vi "设置界面.vi"() -> ()   [LabVIEW 2016, in "DGUS.lvlib"]
uses:
  DGUS.lvlib
  <vilib>/Utility/config.llb/NI_LVConfig.lvlib
panel:
  in  "小数位":u16=2
  in  "底图":enum16{"常规", "摄氏度"}(ring)
  in  "单位":string
  in  "英文名称":string
  in  "中文名称":string
  in  "底部标题":string
  in  "保存按钮":bool
  in  "删除按钮":bool
  in  "添加按钮":bool
  in  "参数列表":i32(listbox)
  # "显示信息设置"
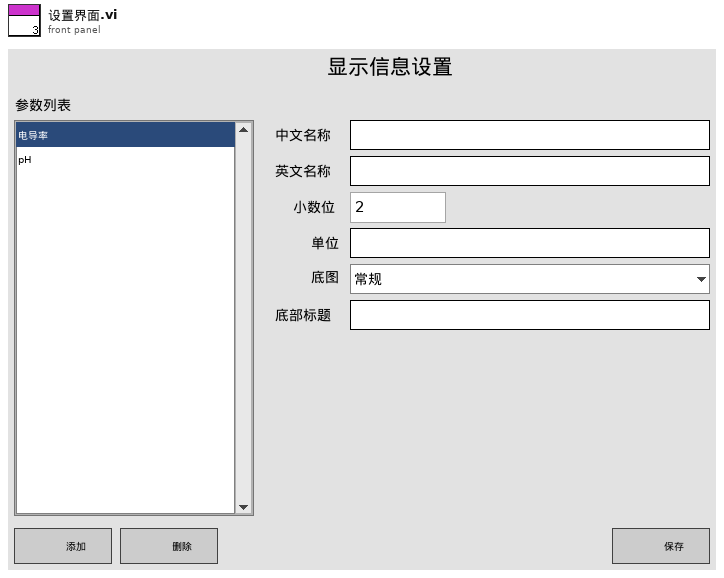
[diagram p1: front panel]
types:
  T1 = typedef "LVPoint32TypeDef.ctl" = cluster{"Horizontal":i32, "Vertical":i32}
  T2 = typedef "NI_LVConfig.lvlib/Config Data RefNum.ctl" = refnum<k1>
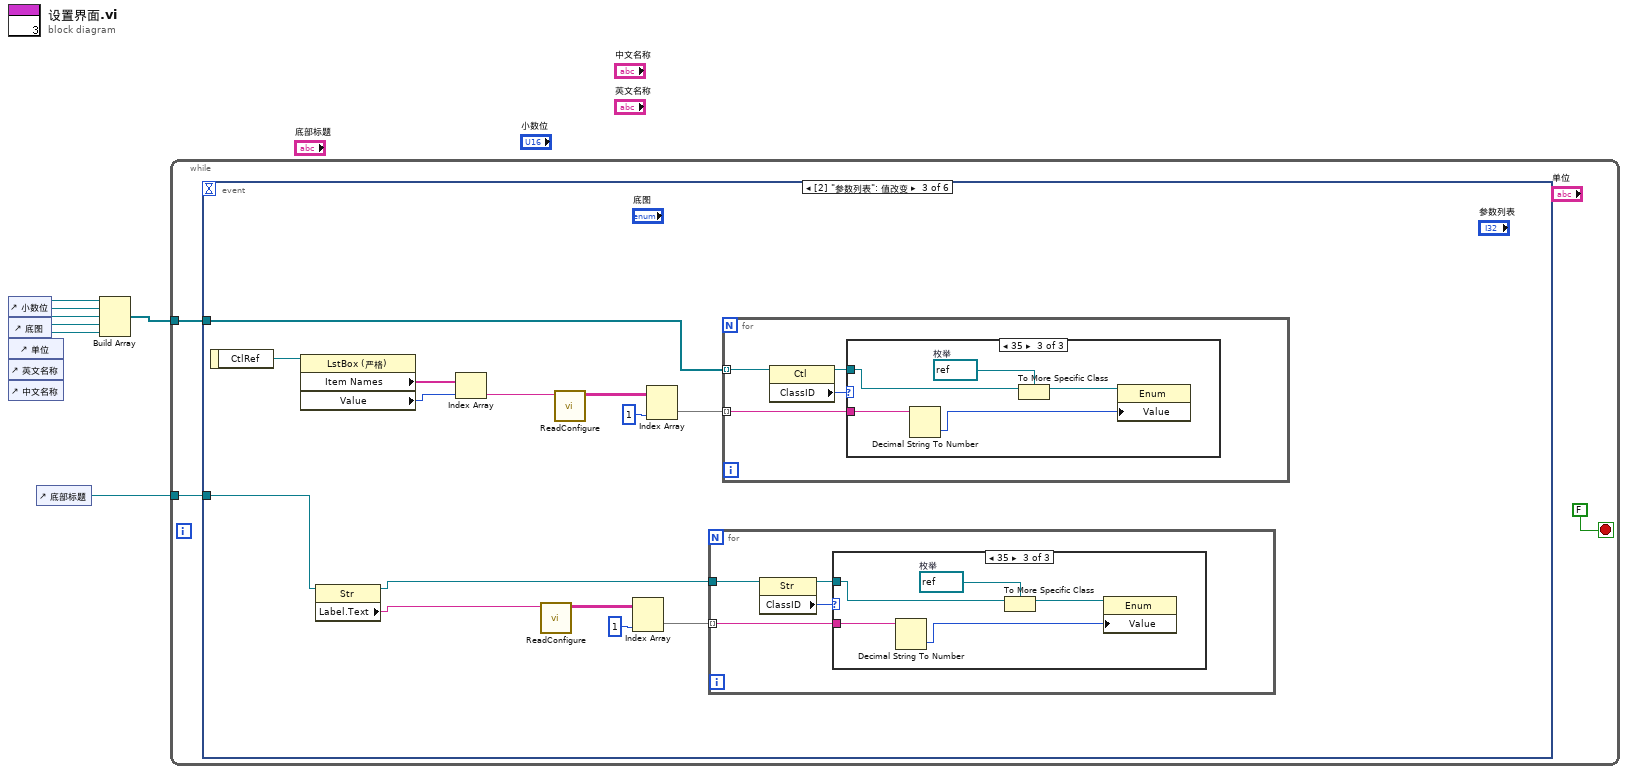
[diagram p0: block diagram]
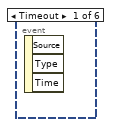
[diagram p2: hidden frame]
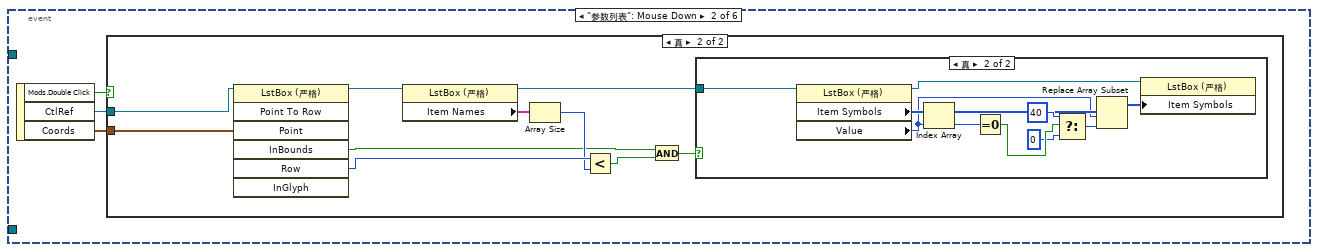
[diagram p3: hidden frame]
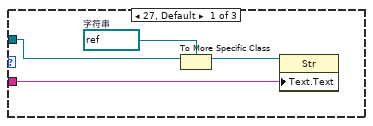
[diagram p6: hidden frame]
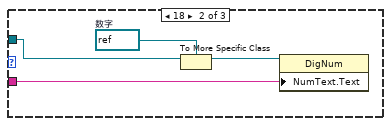
[diagram p7: hidden frame]
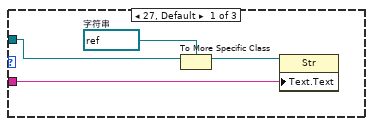
[diagram p8: hidden frame]
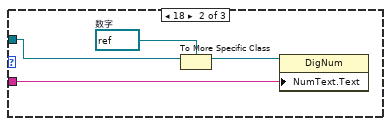
[diagram p9: hidden frame]
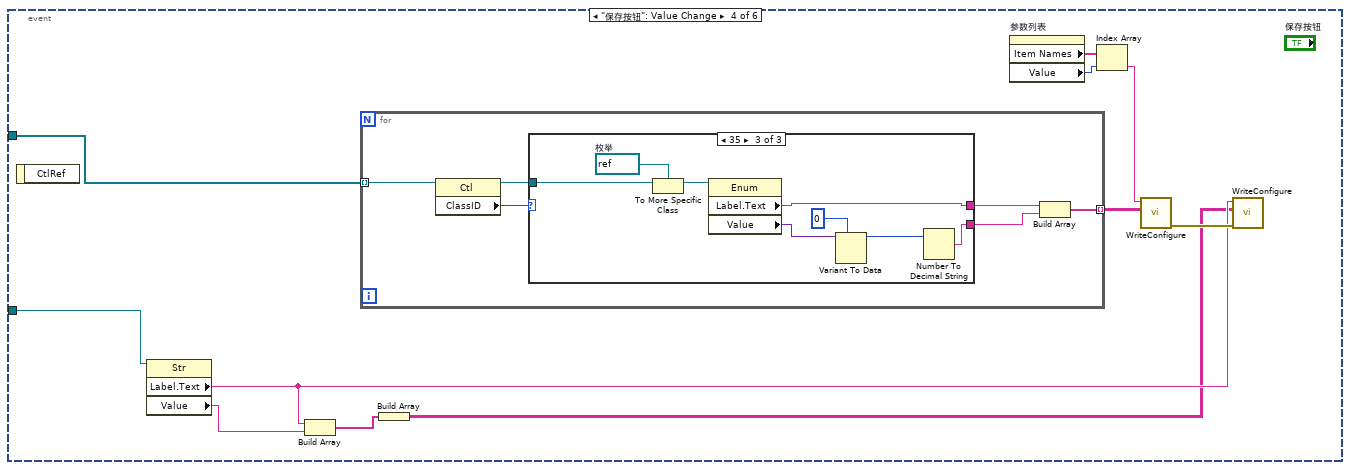
[diagram p10: hidden frame]
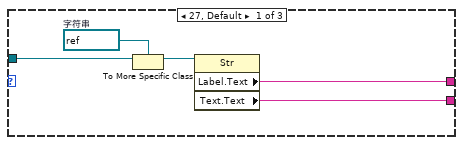
[diagram p11: hidden frame]
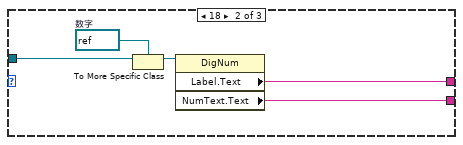
[diagram p12: hidden frame]
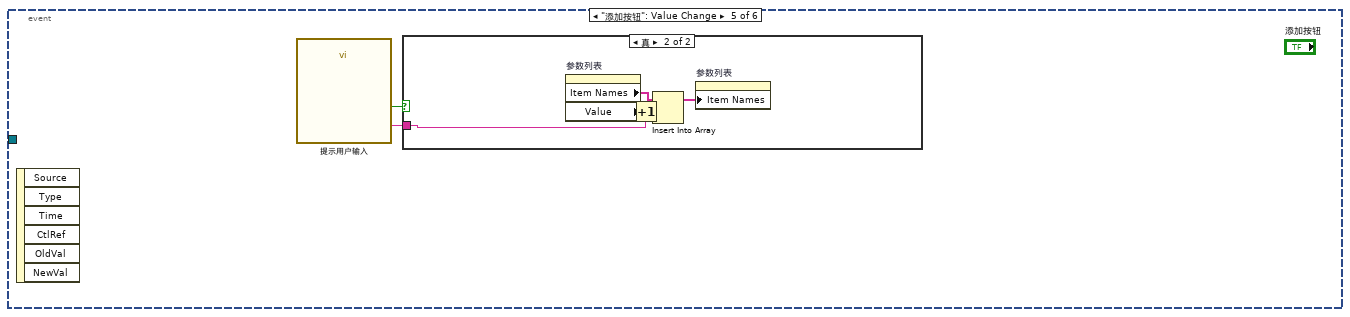
[diagram p13: hidden frame]
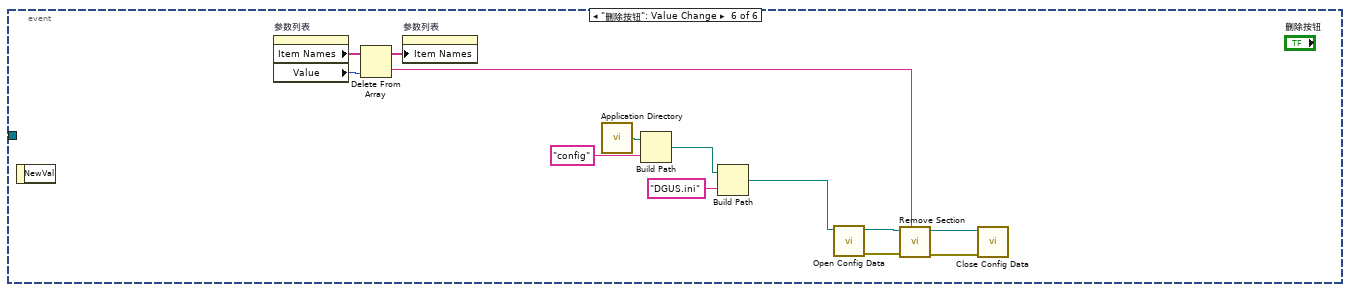
[diagram p15: hidden frame]
diagram:
  n1 = control-ref of="小数位"() -> (w7:refnum<vi>)
  n2 = control-ref of="底图"() -> (w6:refnum<vi>)
  n3 = control-ref of="单位"() -> (w5:refnum<vi>)
  n4 = control-ref of="英文名称"() -> (w4:refnum<vi>)
  n5 = control-ref of="中文名称"() -> (w3:refnum<vi>)
  n6 = control-ref of="底部标题"() -> (w1:refnum<vi>)
  n7 = Build Array(w7, w6, w5, w4, w3) -> (w2:refnum<vi>[])
  n8 = while {
    tunnel: w2 -> [w9]
    tunnel: w1 -> [w8]
    stop <- FALSE stop-if-true
    n9 = event shown="[2] \"参数列表\": 值改变" {
      selector: _ -> [_ _ _ _ _ _]
      dyn-events: _ -> [_ _ _ _ _ _]
      timeout: _ -> [_ _ _ _ _ _]
      tunnel: w9 -> [_ _ w40 w88 _ _]
      tunnel: w8 -> [_ _ w36 w86 _ _]
      event Timeout {
        n10 = event-data() -> ()  [unwired: 1 in, 3 out]
      }
      event "参数列表": Mouse Down {
        n11 = event-data() -> ("Mods.Double Click"=w11:bool, "CtlRef"=w13:refnum<vi>, "Coords"=w12:T1)  [unwired: 1 in]
        n12 = case shown="真" w11 {
          tunnel: w13 -> [_ w23]
          tunnel: w12 -> [_ w21]
          frame False {
          }
          frame True {
            n13 = invoke class="LstBox (严格)" method="Point To Row"(reference=w23, "Point"=w21) -> (reference out=w22:refnum<vi>, "InBounds"=w16:bool, "Row"=w19:i32)  [unwired: 5 in, 4 out]
            n14 = property class="LstBox (严格)"(reference=w22) -> (reference out=w20:refnum<vi>, "Item Names"=w18:string[])  [unwired: 1 in, 1 out]
            n15 = Array Size(array=w18) -> (size(s)=w17:i32)
            n16 = Less?(x=w19, y=w17) -> (x < y?=w15:bool)
            n17 = And(x=w16, y=w15) -> (x .and. y?=w14:bool)
            n18 = case shown="真" w14 {
              tunnel: w20 -> [_ w24]
              frame False {
              }
              frame True {
                n19 = property class="LstBox (严格)"(reference=w24) -> (reference out=w26:refnum<vi>, "Item Symbols"=w29:i32[], "Value"=w28:i32)  [unwired: 1 in, 1 out]
                n20 = Index Array(array=w29, index=w28) -> (element=w33:i32)
                n21 = Equal To 0?(x=w33) -> (x = 0?=w32:bool)
                n22 = Select(t=40, s=w32, f=0) -> (s? t:f=w27:i32)
                n23 = Replace Array Subset(array=w29, new element=w27, index=w28) -> (w25:i32[])
                n24 = property class="LstBox (严格)"(reference=w26, "Item Symbols"=w25) -> ()  [unwired: 1 in, 2 out]
              }
            }
          }
        }
      }
      event "参数列表": Value Change {
        n25 = event-data() -> ("CtlRef"=w44:refnum<vi>)  [unwired: 1 in]
        n26 = property class="LstBox (严格)"(reference=w44) -> ("Item Names"=w43:string[], "Value"=w42:i32)  [unwired: 1 in, 2 out]
        n27 = property class="Str"(reference=w36) -> (reference out=w34:refnum<vi>, "Label.Text"=w35:string)  [unwired: 1 in, 1 out]
        n28 = Index Array(array=w43, index=w42) -> (element=w41:string)
        n29 = call "ReadConfigure.vi"("section"=w35) -> ("Para"=w38:string[][])  [unwired: 9 in, 1 out]
        n30 = call "ReadConfigure.vi"("section"=w41) -> ("Para"=w46:string[][])  [unwired: 9 in, 1 out]
        n31 = Index Array(array=w38, index (col)=1 ("禁用的索引 (列)")) -> (element=w37:string[])  [unwired: 1 in]
        n32 = Index Array(array=w46, index (col)=1 ("禁用的索引 (列)")) -> (element=w47:string[])  [unwired: 1 in]
        n33 = for {
          tunnel: w34 -> [w51]
          tunnel: w37 -> [w48] mode=indexing
          n34 = property class="Str"(reference=w51) -> (reference out=w49:refnum<vi>, "ClassID"=w50:u32)  [unwired: 1 in, 1 out]
          n35 = case shown="35" w50 {
            tunnel: w49 -> [w55 w59 w64]
            tunnel: w48 -> [w52 w56 w61]
            frame 27, Default {
              w54 = refnum<vi> refnum  # 字符串
              n36 = To More Specific Class(target class=w54, reference=w55) -> (specific class reference=w53:refnum<vi>)  [unwired: 1 in, 1 out]
              n37 = property class="Str"(reference=w53, "Text.Text"=w52) -> ()  [unwired: 1 in, 2 out]
            }
            frame 18 {
              w58 = refnum<vi> refnum  # 数字
              n38 = To More Specific Class(target class=w58, reference=w59) -> (specific class reference=w57:refnum<vi>)  [unwired: 1 in, 1 out]
              n39 = property class="DigNum"(reference=w57, "NumText.Text"=w56) -> ()  [unwired: 1 in, 2 out]
            }
            frame 35 {
              w63 = refnum<vi> refnum  # 枚举
              n40 = Decimal String To Number(string=w61) -> (number=w60:i32)  [unwired: 2 in, 1 out]
              n41 = To More Specific Class(target class=w63, reference=w64) -> (specific class reference=w62:refnum<vi>)  [unwired: 1 in, 1 out]
              n42 = property class="Enum"(reference=w62, "Value"=w60) -> ()  [unwired: 1 in, 2 out]
            }
          }
        }
        n43 = for {
          tunnel: w40 -> [w68] mode=indexing
          tunnel: w47 -> [w65] mode=indexing
          n44 = property class="Ctl"(reference=w68) -> (reference out=w66:refnum<vi>, "ClassID"=w67:u32)  [unwired: 1 in, 1 out]
          n45 = case shown="35" w67 {
            tunnel: w66 -> [w72 w76 w81]
            tunnel: w65 -> [w69 w73 w78]
            frame 27, Default {
              w71 = refnum<vi> refnum  # 字符串
              n46 = To More Specific Class(target class=w71, reference=w72) -> (specific class reference=w70:refnum<vi>)  [unwired: 1 in, 1 out]
              n47 = property class="Str"(reference=w70, "Text.Text"=w69) -> ()  [unwired: 1 in, 2 out]
            }
            frame 18 {
              w75 = refnum<vi> refnum  # 数字
              n48 = To More Specific Class(target class=w75, reference=w76) -> (specific class reference=w74:refnum<vi>)  [unwired: 1 in, 1 out]
              n49 = property class="DigNum"(reference=w74, "NumText.Text"=w73) -> ()  [unwired: 1 in, 2 out]
            }
            frame 35 {
              w80 = refnum<vi> refnum  # 枚举
              n50 = Decimal String To Number(string=w78) -> (number=w77:i32)  [unwired: 2 in, 1 out]
              n51 = To More Specific Class(target class=w80, reference=w81) -> (specific class reference=w79:refnum<vi>)  [unwired: 1 in, 1 out]
              n52 = property class="Enum"(reference=w79, "Value"=w77) -> ()  [unwired: 1 in, 2 out]
            }
          }
        }
      }
      event "保存按钮": Value Change {
        n53 = event-data() -> ()  [unwired: 1 in, 1 out]
        n54 = property class="Str"(reference=w86) -> ("Label.Text"=w85:string, "Value"=w84:string)  [unwired: 1 in, 2 out]
        n55 = Build Array(w85, w84) -> (w83:string[])
        n56 = for {
          tunnel: w88 -> [w98] mode=indexing
          tunnel: [w93] -> w89 mode=indexing
          n57 = property class="Ctl"(reference=w98) -> (reference out=w96:refnum<vi>, "ClassID"=w97:u32)  [unwired: 1 in, 1 out]
          n58 = case shown="35" w97 {
            tunnel: w96 -> [w103 w108 w116]
            tunnel: [w100 w105 w113] -> w95
            tunnel: [w99 w104 w109] -> w94
            frame 27, Default {
              w102 = refnum<vi> refnum  # 字符串
              n59 = To More Specific Class(target class=w102, reference=w103) -> (specific class reference=w101:refnum<vi>)  [unwired: 1 in, 1 out]
              n60 = property class="Str"(reference=w101) -> ("Label.Text"=w100:string, "Text.Text"=w99:string)  [unwired: 1 in, 2 out]
            }
            frame 18 {
              w107 = refnum<vi> refnum  # 数字
              n61 = To More Specific Class(target class=w107, reference=w108) -> (specific class reference=w106:refnum<vi>)  [unwired: 1 in, 1 out]
              n62 = property class="DigNum"(reference=w106) -> ("Label.Text"=w105:string, "NumText.Text"=w104:string)  [unwired: 1 in, 2 out]
            }
            frame 35 {
              w115 = refnum<vi> refnum  # 枚举
              n63 = To More Specific Class(target class=w115, reference=w116) -> (specific class reference=w114:refnum<vi>)  [unwired: 1 in, 1 out]
              n64 = property class="Enum"(reference=w114) -> ("Label.Text"=w113:string, "Value"=w112:variant)  [unwired: 1 in, 2 out]
              n65 = Variant To Data(type=0, Variant=w112) -> (data=w110:i32)  [unwired: 1 in, 1 out]
              n66 = Number To Decimal String(number=w110) -> (decimal integer string=w109:string)  [unwired: 1 in]
            }
          }
          n67 = Build Array(w95, w94) -> (w93:string[])
        }
        n68 = Build Array(w83) -> (w82:string[][])
        n69 = property on="参数列表" class="LstBox (严格)"() -> ("Item Names"=w92:string[], "Value"=w91:i32)  [unwired: 2 in, 2 out]
        n70 = Index Array(array=w92, index=w91) -> (element=w90:string)
        n71 = call "WriteConfigure.vi"("Para"=w89, "section"=w90) -> ("error out"=w87:errorcluster)  [unwired: 9 in]
        n72 = call "WriteConfigure.vi"("error in (no error)"=w87, "Para"=w82, "section"=w85) -> ()  [unwired: 8 in, 1 out]
      }
      event "添加按钮": Value Change {
        n73 = event-data() -> ()  [unwired: 1 in, 6 out]
        n74 = call "提示用户输入"() -> ("参数名称"=w118:string, "确定"=w117:bool)  [unwired: 17 in, 1 out]
        n75 = case shown="真" w117 {
          tunnel: w118 -> [_ w120]
          frame False {
          }
          frame True {
            n76 = property on="参数列表" class="LstBox (严格)"() -> ("Item Names"=w123:string[], "Value"=w121:i32)  [unwired: 2 in, 2 out]
            n77 = Increment(x=w121) -> (x+1=w119:i32)
            n78 = Insert Into Array(array=w123, index=w119, new element=w120) -> (w122:string[])
            n79 = property on="参数列表" class="LstBox (严格)"("Item Names"=w122) -> ()  [unwired: 2 in, 2 out]
          }
        }
      }
      event "删除按钮": Value Change {
        n80 = event-data() -> ()  [unwired: 1 in, 1 out]
        n81 = property on="参数列表" class="LstBox (严格)"() -> ("Item Names"=w136:string[], "Value"=w135:i32)  [unwired: 2 in, 2 out]
        n82 = Delete From Array(array=w136, index=w135) -> (deleted portion=w127:string, array with subset deleted=w134:string[])  [unwired: 1 in]
        n83 = property on="参数列表" class="LstBox (严格)"("Item Names"=w134) -> ()  [unwired: 2 in, 2 out]
        n84 = call <vilib>:"Application Directory.vi"() -> ("Application Directory"=w133:path)
        n85 = Build Path(base path=w133, name or relative path="config" ("名称或相对路径")) -> (appended path=w131:path)
        n86 = Build Path(base path=w131, name or relative path="DGUS.ini" ("名称或相对路径")) -> (appended path=w129:path)
        n87 = call <vilib>:"Open Config Data.vi"("configuration file path"=w129) -> ("error out"=w126:errorcluster, "refnum"=w128:T2)  [unwired: 8 in, 1 out]
        n88 = call <vilib>:"Remove Section.vi"("section"=w127, "error in (no error)"=w126, "refnum"=w128) -> ("error out"=w124:errorcluster, "refnum out"=w125:T2)  [unwired: 6 in, 1 out]
        n89 = call <vilib>:"Close Config Data.vi"("error in (no error)"=w124, "refnum"=w125) -> ()  [unwired: 8 in, 2 out]
      }
    }
  }
